vi "demo-testflow.vi"(11 "Message Cluster":T1) -> (3 "Message Cluster 2":T1)   [LabVIEW 2017]
uses:
  Message Queue/Message Cluster.ctl
  Message Queue/Message Queue.lvlib
  <vilib>/Instr/_visa.llb/VISA Configure Serial Port (Instr).vi
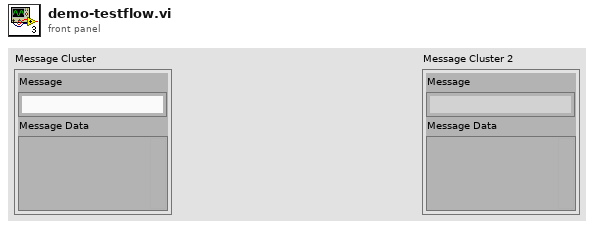
[diagram p1: front panel]
types:
  T1 = typedef "Message Queue.lvlib/Message Cluster.ctl" = cluster{"Message":string, "Message Data":variant}
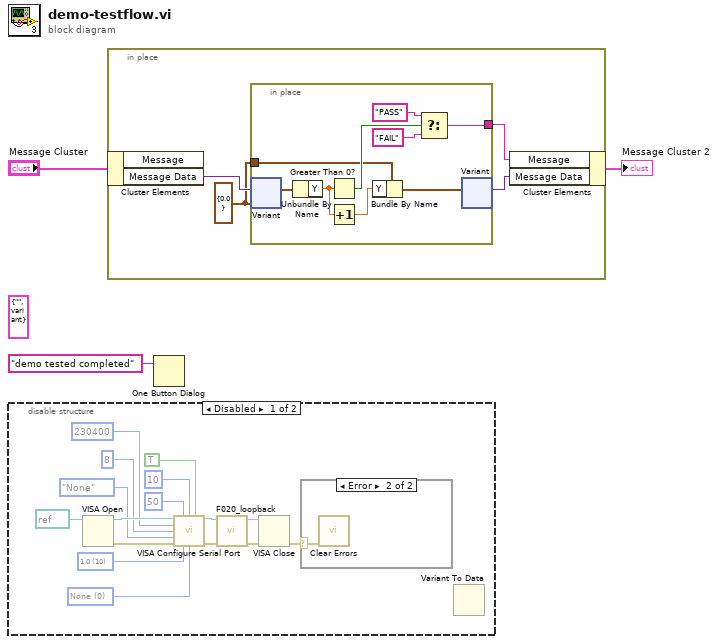
[diagram p0: block diagram]
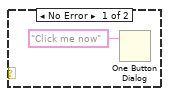
[diagram p2: hidden frame]
diagram:
  (unwired) T1 {"Message"="", "Message Data"=variant} ("Message Cluster")
  n1 = disable-structure shown="Disabled" {
    frame Disabled {
      w12 = u16 10 items=["1.0"=10, "1.5"=15, "2.0"=20] ("stop bits (10: 1 bit)")
      w11 = u16 0 items=["None", "XON/XOFF", "RTS/CTS", "XON/XOFF & RTS/CTS", "DTR/DSR", "XON/XOFF & DTR/DSR"] ("flow control (0:none)")
      n2 = VISA Open(VISA resource name=refnum<visa-resource-name> refnum) -> (VISA resource name=w19:refnum<visa-resource-name>, error out=w18:errorcluster)  [unwired: 4 in]
      n3 = call-poly "VISA Configure Serial Port"("VISA resource name"=w19, "timeout (10sec)"=u32 50, "termination char\n(0xA = '\\n' = LF)"=u32 10 ("timeout (10sec)"), "Enable Termination\nChar (T)"=TRUE ("Enable Termination\nChar (T)"), "baud rate (9600)"=u64 230400 ("Baud rate"), "data bits (8)"=u16 8, "parity (0:none)"=enum16{"None", "Odd", "Even", "Mark", "Space"}."None", "error in (no error)"=w18, "stop bits (10: 1 bit)"=w12, "flow control (0:none)"=w11) -> ("VISA resource name out"=w8:refnum<visa-resource-name>, "error out"=w7:errorcluster)  [unwired: 4 in]
      n4 = call "F020_loopback.vi"("error in"=w7, "COM in"=w8) -> ("error out"=w5:errorcluster, "COM out"=w6:string)  [unwired: 8 in]
      n5 = VISA Close(VISA resource name=w6, error in (no error)=w5) -> (error out=w4:errorcluster)
      n6 = case shown="Error" w4 {
        selector: w4 -> [_ w21]
        frame No Error {
          n7 = One Button Dialog(message="Click me now") -> ()  [unwired: 1 in, 1 out]
        }
        frame Error {
          n8 = call <vilib>:"Clear Errors.vi"("error in (no error)"=w21) -> ()  [unwired: 5 in, 2 out]
        }
      }
      n9 = Variant To Data() -> ()  [unwired: 3 in, 2 out]
    }
    frame Enabled {
    }
  }
  n10 = in-place {
    w24 = cluster{"Y":dbl} {"Y"=0.0} ("output cluster")
    n11 = in-place-cluster #1("Message Cluster") -> ("Message Data"=w25:variant)  [unwired: 1 out]
    n12 = in-place {
      in-place-border: [w31] -> w22
      in-place-border: w24 -> [w26]
      n13 = in-place-variant #2(w25, w24) -> (w28:cluster{"Y":dbl})  [unwired: 1 out]
      n14 = Unbundle By Name(w28) -> ("Y"=w29:dbl)
      n15 = Greater Than 0?(x=w29) -> (x > 0?=w30:bool)
      n16 = Increment(x=w29) -> (x+1=w34:dbl)
      n17 = Bundle By Name(cluster=w26, "Y"=w34) -> (w27:cluster{"Y":dbl})
      n18 = Select(t="PASS" ("Message"), s=w30, f="FAIL") -> (s? t:f=w31:string)
      n19 = in-place-variant #2(w27) -> (w23:variant)  [unwired: 1 out]
    }
    n20 = in-place-cluster #1("Message"=w22, "Message Data"=w23) -> (→"Message Cluster 2":T1)
  }
  n21 = One Button Dialog(message="demo tested completed") -> ()  [unwired: 1 in, 1 out]
